vi "PXF4_init_param.vi"(8 "error in":errorcluster, 11 "Modbus Master in":refnum<class "Modbus Master.lvclass">) -> (0 "error out":errorcluster, 3 "Modbus Master out":refnum<class "Modbus Master.lvclass">)   [LabVIEW 2019]
uses:
  <vilib>/NI/Modbus Library/API/Master/Modbus Master.lvclass
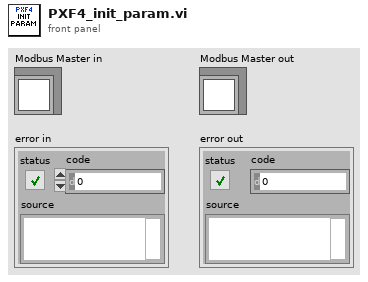
[diagram p1: front panel]
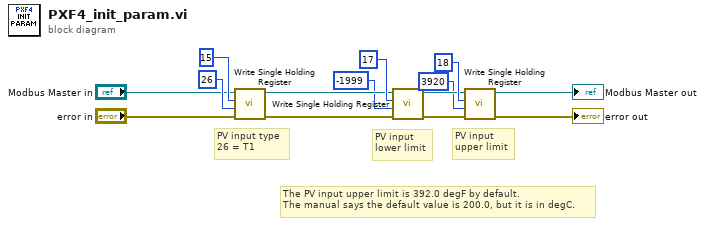
[diagram p0: block diagram]
diagram:
  # "The PV input upper limit is 392.0 degF by default.\nThe manual says the default value is 200.0, but it is in degC."
  # "PV input \nupper limit"
  # "PV input \nlower limit"
  # "PV input type\n26 = T1"
  n1 = call-dynamic "Write Single Holding Register.vi"("error in"="error in", "register to write"=u16 26, "address"=u16 15, "Modbus master in"="Modbus Master in") -> ("error out"=w9:errorcluster, "Modbus master out"=w7:refnum<class "Modbus Master.lvclass">)  [unwired: 6 in]
  n2 = call-dynamic "Write Single Holding Register.vi"("error in"=w9, "register to write"=i16 -1999, "address"=u16 17, "Modbus master in"=w7) -> ("error out"=w10:errorcluster, "Modbus master out"=w8:refnum<class "Modbus Master.lvclass">)  [unwired: 6 in]
  n3 = call-dynamic "Write Single Holding Register.vi"("error in"=w10, "register to write"=u16 3920, "address"=u16 18, "Modbus master in"=w8) -> ("error out"=→"error out":errorcluster, "Modbus master out"=→"Modbus Master out":refnum<class "Modbus Master.lvclass">)  [unwired: 6 in]
